vi "SUB-칼만 필터_IMU.vi"(3 "x set":dbl[](array[numeric]) step=1.0) -> (1 "Kalman X":dbl[](array[numeric]) format="%.5f")   [LabVIEW 2015]
panel:
  out "P":dbl[](array[numeric])
  out "x":dbl[](array[numeric])
  # "칼만 필터"
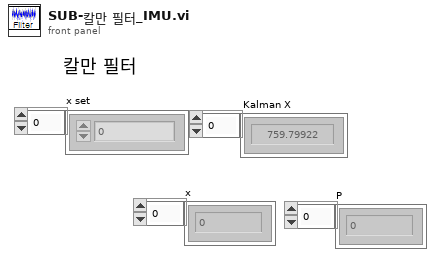
[diagram p1: front panel]
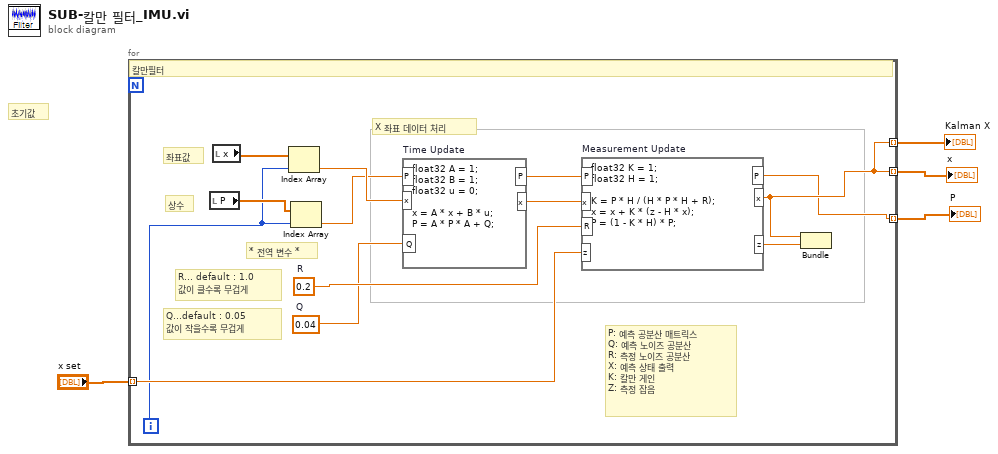
[diagram p0: block diagram]
diagram:
  # "초기값"
  n1 = for {
    tunnel: "x set" -> [w12] mode=indexing
    tunnel: [w11] -> w3 mode=indexing
    tunnel: [w11] -> w2 mode=indexing
    tunnel: [w10] -> w1 mode=indexing
    i -> [w5]
    w16 = 0.04  # Q
    w17 = 0.2  # R
    # "좌표값"
    # "상수"
    # "P: 예측 공분산 매트릭스\nQ: 예측 노이즈 공분산\nR: 측정 노이즈 공분산\nX: 예측 상태 출력 \nK: 칼만 게인\nZ: 측정 잡음"
    # "X 좌표 데이터 처리"
    # "* 전역 변수 *"
    # "Q...default : 0.05\n값이 작을수록 무겁게"
    # "R... default : 1.0\n값이 클수록 무겁게"
    # "칼만필터"
    n2 = local read "P"() -> (w6:dbl[])
    n3 = local read "x"() -> (w9:dbl[])
    n4 = Index Array(array=w9, index=w5) -> (element=w8:dbl)
    n5 = Index Array(array=w6, index=w5) -> (element=w7:dbl)
    n6 = formula code="float32 A = 1;\nfloat32 B = 1;\nfloat32 u = 0;\n\nx = A * x + B * u;\nP = A * P * A + Q;" "Time Update"("x"=w8, "P"=w7, "Q"=w16) -> ("x"=w15:dbl, "P"=w14:dbl)
    n7 = formula code="float32 K = 1;\nfloat32 H = 1;\n\nK = P * H / (H * P * H + R);\nx = x + K * (z - H * x);\nP = (1 - K * H) * P;" "Measurement Update"("x"=w15, "P"=w14, "z"=w12, "R"=w17) -> ("x"=w11:dbl, "P"=w10:dbl, "z"=w13:dbl)
    n8 = Bundle("x"=w11, "z"=w13) -> ()  [unwired: 1 in, 1 out]
  }
  "Kalman X" <- w3
  "x" <- w2
  "P" <- w1
